vi "Write Hardware Handles.vi"(8 "error in":errorcluster, 10 "hardware handles":T1, 11 "Ballard ARINC-429 Execution Unit in":refnum<class "Execution Unit.lvclass">) -> (0 "error out":errorcluster, 3 "Ballard ARINC-429 Execution Unit out":refnum<class "Execution Unit.lvclass">)   [LabVIEW 2020, in "AIM ARINC 429 Engine.lvlib" / "Implementation.lvlib" / "Execution Unit.lvclass"]
uses:
  Execution Unit.lvclass
  Custom Device/Hardware Handles.ctl
  Execution Unit.lvclass/Execution Unit.ctl
  Custom Device/Custom Device.lvlib
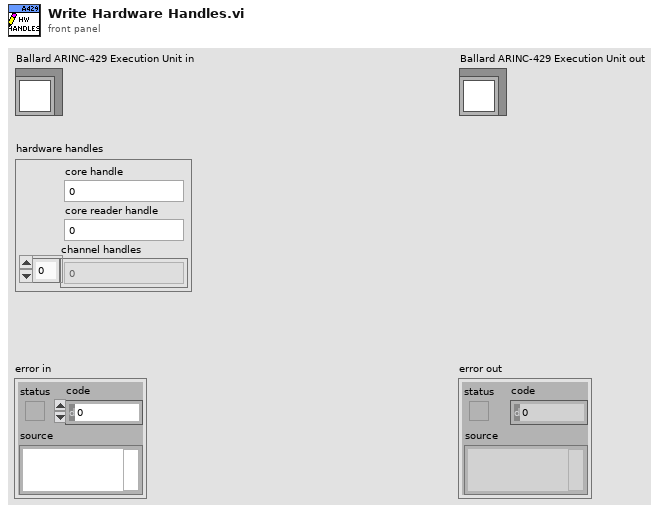
[diagram p1: front panel]
types:
  T1 = typedef "AIM ARINC 429 Engine.lvlib/Custom Device.lvlib/Hardware Handles.ctl" = cluster{"core handle":u64, "core reader handle":u64, "channel handles":u64[]}
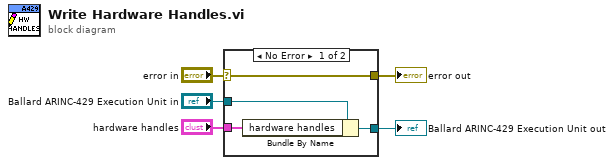
[diagram p0: block diagram]
diagram:
  n1 = case shown="No Error" "error in" {
    selector: "error in" -> [w9 w10]
    tunnel: [w9 w10] -> w4
    tunnel: [w7 w11] -> w2
    tunnel: "Ballard ARINC-429 Execution Unit in" -> [w8 w11]
    tunnel: "hardware handles" -> [w6 _]
    frame No Error {
      n2 = Bundle By Name(cluster=w8, "hardware handles"=w6) -> (w7:refnum<class "Execution Unit.lvclass">)
    }
    frame Error {
    }
  }
  "error out" <- w4
  "Ballard ARINC-429 Execution Unit out" <- w2
